vi "Advance Settings UI.vi"(0 "Advance Setting In":T1={"Prepare"={"Power Test Board.Voltage Level (V)"=0.0, "Power Test Board.Current Limit (A)"=0.0, "Fgen Voltage to Current Ratio"=1.0, "Fgen.Sample Rate (Sample/s)"=1.0}, "Stimulus And Measure"={"Fgen.Offset (V)"=0.0}} {"Stimulus And Measure"."Fgen.Offset (V)" min=1.0 format="%#_6p"; "Prepare"."Power Test Board.Current Limit (A)" min=1.0 format="%#_6p"; "Prepare"."Power Test Board.Voltage Level (V)" min=1.0 format="%#_6p"; "Prepare"."Fgen.Sample Rate (Sample/s)" min=1.0 format="%#_6p"; "Prepare"."Fgen Voltage to Current Ratio" min=1.0 format="%#_6p"}, 11 "error in (no error)":errorcluster) -> (4 "Advance Setting Out":T1={"Prepare"={"Power Test Board.Voltage Level (V)"=0.0, "Power Test Board.Current Limit (A)"=0.0, "Fgen Voltage to Current Ratio"=1.0, "Fgen.Sample Rate (Sample/s)"=1.0}, "Stimulus And Measure"={"Fgen.Offset (V)"=0.0}} {"Stimulus And Measure"."Fgen.Offset (V)" min=1.0 format="%#_6p"; "Prepare"."Power Test Board.Current Limit (A)" min=1.0 format="%#_6p"; "Prepare"."Power Test Board.Voltage Level (V)" min=1.0 format="%#_6p"; "Prepare"."Fgen.Sample Rate (Sample/s)" min=1.0 format="%#_6p"; "Prepare"."Fgen Voltage to Current Ratio" min=1.0 format="%#_6p"}, 15 "error out":errorcluster)   [LabVIEW 2020, in "LDO Load Transient_AWG.lvlib"]
uses:
  LDO Load Transient_AWG.lvlib
  Typedefs/Advance Settings.ctl
  Typedefs/Adv Settings Setup Instr.ctl
  Typedefs/Adv Settings Stimulus and Measure.ctl
  <vilib>/Utility/error.llb/DialogType.ctl
  <userlib>/_Soliton/Measurement Suite/Reusables/Queue Driver/Plugin Queue Driver.lvlib
  <userlib>/_Soliton/Measurement Suite/Reusables/Plugin Common/Plugin Common.lvlib
panel:
  in  "Current Limit (A)":dbl=0.1 min=1.0 format="%#_6p"
  in  "Voltage Level (V)":dbl=6.0 min=1.0 format="%#_6p"
  in  "Offset (V)":dbl min=1.0 format="%#_6p"
  in  "Sample Rate (Sample/s)":dbl=20000000.0 min=1.0 format="%#_6p"
  in  "Fgen Voltage to Current Ratio":dbl=1.0 min=1.0 format="%#_6p"
  in  "CLOSE":bool
  in  "Panel Close":bool
  out "Banner":picture caption="Advance Settings"
  # "Power Test Board"
  # "Fgen"
  # "Fgen"
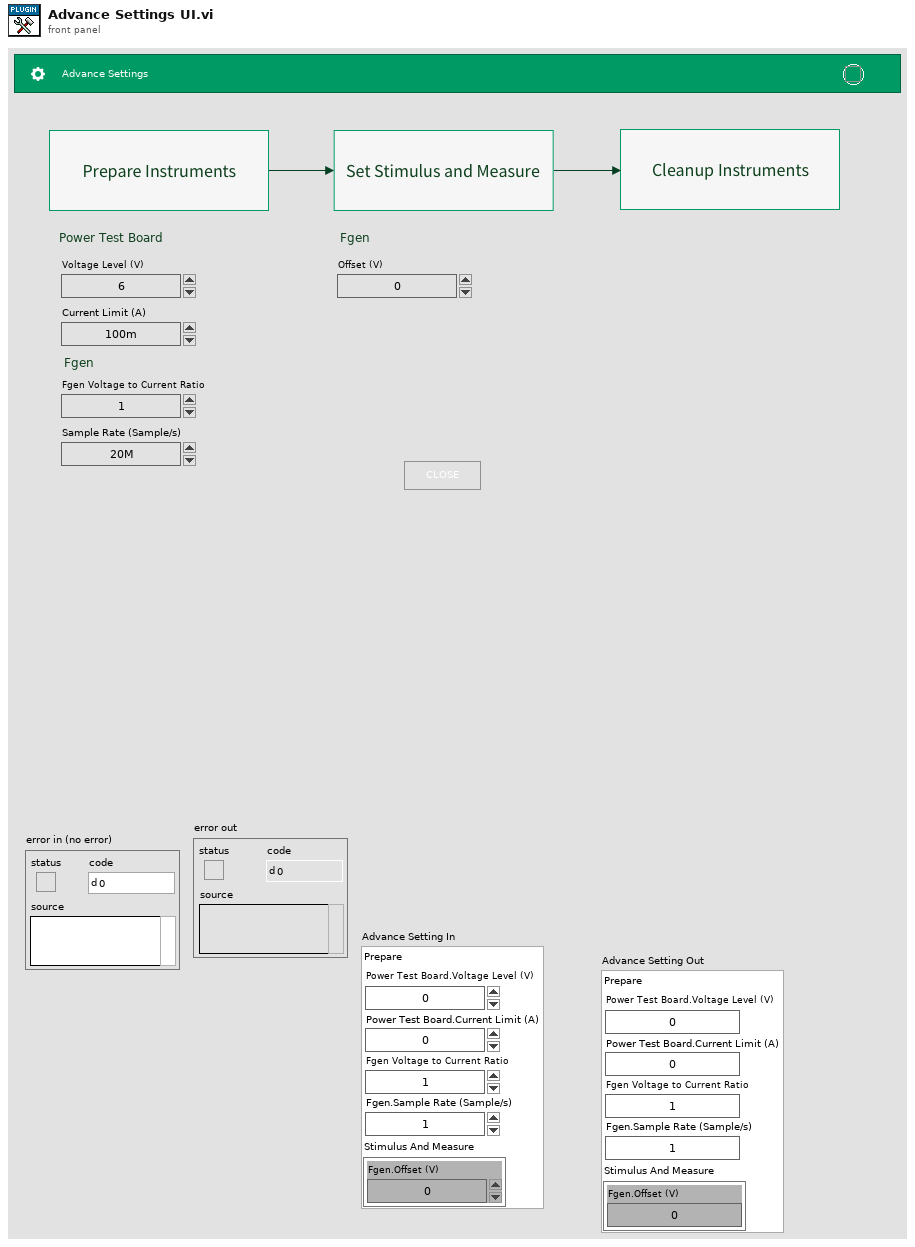
[diagram p1: front panel]
types:
  T1 = typedef "LDO Load Transient_AWG.lvlib/Advance Settings.ctl" = cluster{"Prepare":T2, "Stimulus And Measure":T3}
  T2 = typedef "LDO Load Transient_AWG.lvlib/Adv Settings Setup Instr.ctl" = cluster{"Power Test Board.Voltage Level (V)":dbl, "Power Test Board.Current Limit (A)":dbl, "Fgen Voltage to Current Ratio":dbl, "Fgen.Sample Rate (Sample/s)":dbl}
  T3 = typedef "LDO Load Transient_AWG.lvlib/Adv Settings Stimulus and Measure.ctl" = cluster{"Fgen.Offset (V)":dbl}
  T4 = typedef "DialogType.ctl" = u16
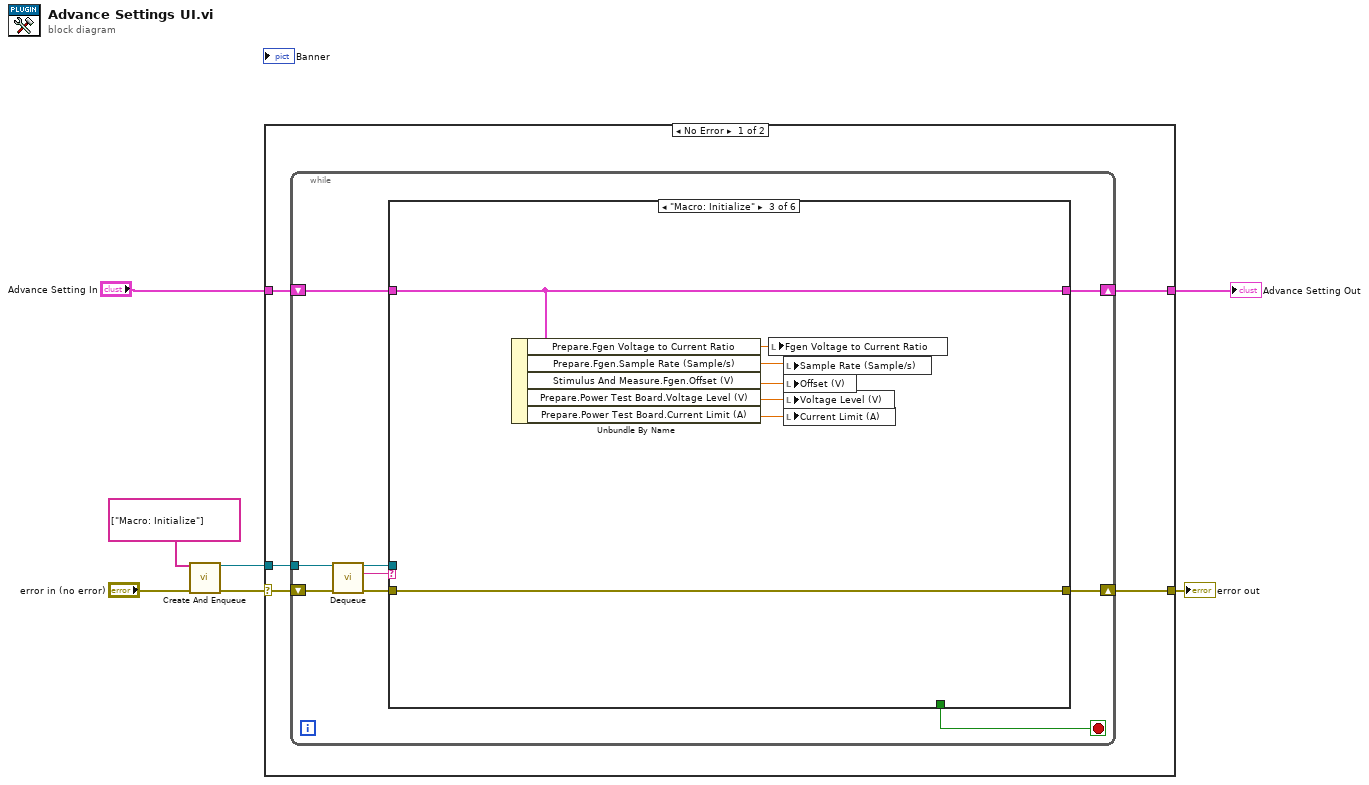
[diagram p0: block diagram]
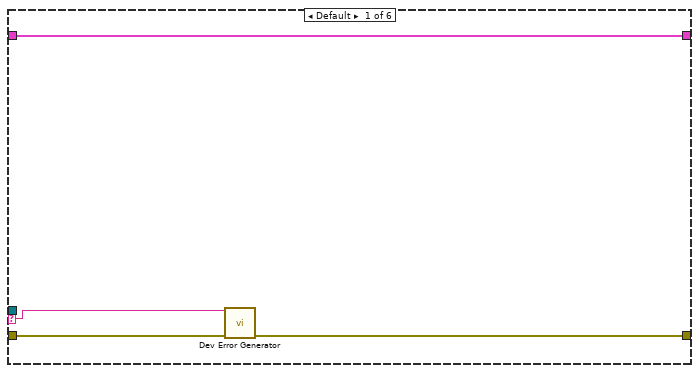
[diagram p2: hidden frame]
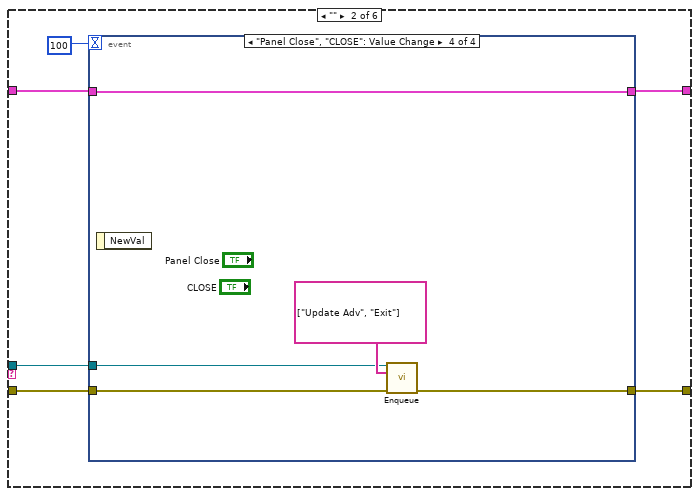
[diagram p3: hidden frame]
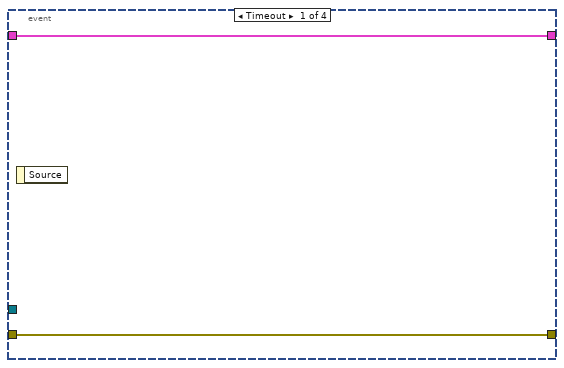
[diagram p4: hidden frame]
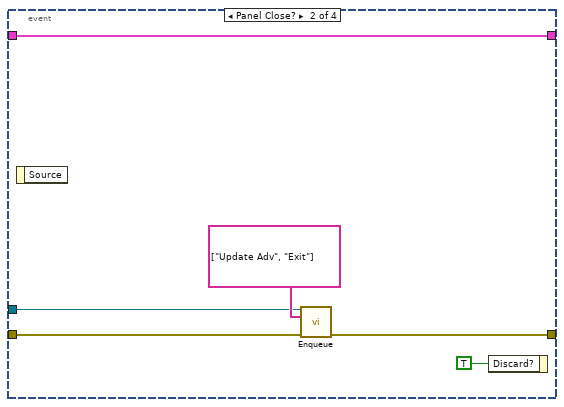
[diagram p5: hidden frame]
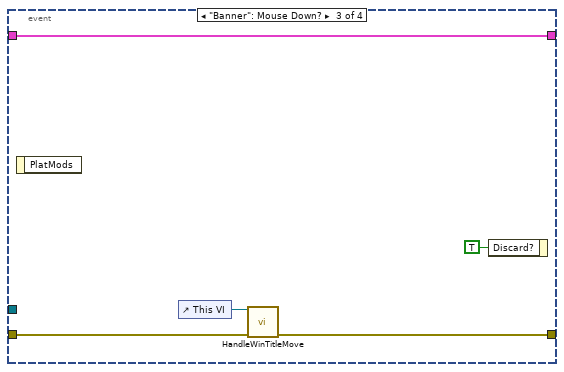
[diagram p6: hidden frame]
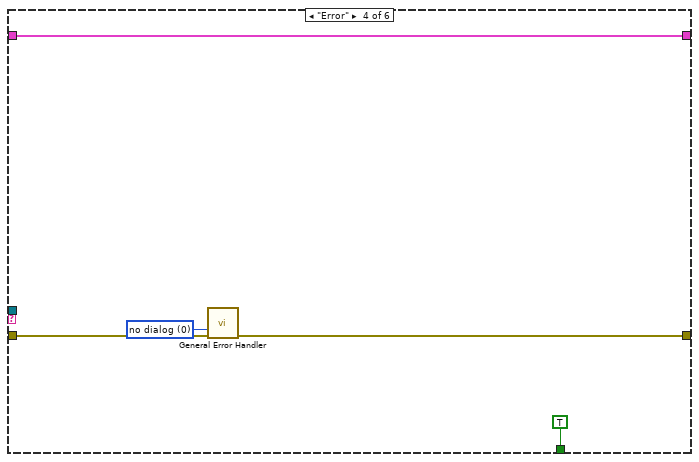
[diagram p7: hidden frame]
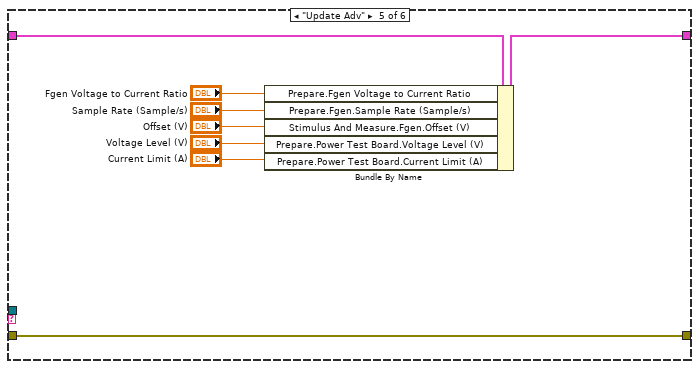
[diagram p8: hidden frame]
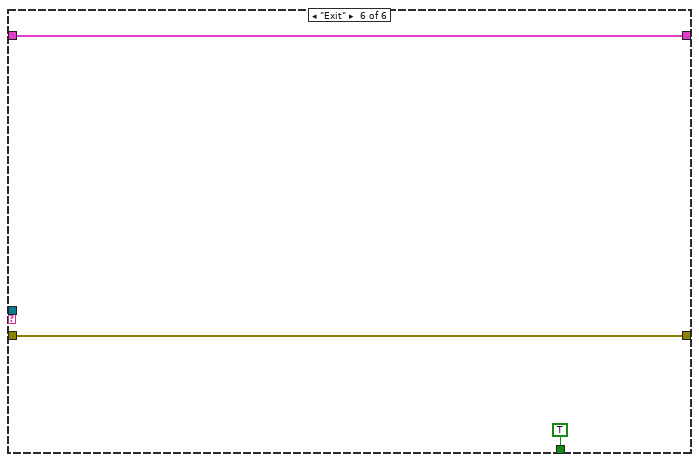
[diagram p9: hidden frame]
diagram:
  n1 = call <userlib>:"Create And Enqueue.vi"("Initial States"=string[] ["Macro: Initialize"], "error in (no error)"="error in (no error)") -> ("Queue out"=w4:refnum<queue>, "error out"=w5:errorcluster)  [unwired: 12 in]
  n2 = case shown="No Error" w5 {
    selector: w5 -> [w8 w74]
    tunnel: [w12 w74] -> w7
    tunnel: "Advance Setting In" -> [w11 w73]
    tunnel: [w10 w73] -> w1
    tunnel: w4 -> [w9 _]
    frame No Error {
      n3 = while {
        tunnel: w9 -> [w18]
        shift-right: [w19] -> w10
        shift-left: w11 -> [w20]
        shift-right: [w21] -> w12
        shift-left: w8 -> [w17]
        stop <- w14 stop-if-true
        n4 = call <userlib>:"Dequeue.vi"("Queue in"=w18, "error in (no error)"=w17) -> ("Queue out"=w13:refnum<queue>, "Dequeued State"=w15:string, "error out"=w16:errorcluster)  [unwired: 11 in]
        n5 = case shown="\"Macro: Initialize\"" w15 {
          selector: w15 -> [w22 _ _ _ _ _]
          tunnel: [w24 w31 w56 w59 w69 w72] -> w21
          tunnel: w20 -> [w25 w30 w55 w61 w67 w71]
          tunnel: [w25 w29 w55 w61 w68 w71] -> w19
          tunnel: w16 -> [w23 w28 w56 w58 w69 w72]
          tunnel: [_ _ _ TRUE _ TRUE ("Discard?")] -> w14
          tunnel: w13 -> [_ w26 _ _ _ _]
          frame Default {
            n6 = call <userlib>:"Dev Error Generator.vi"("State"=w22, "error in (no error)"=w23) -> ("error out"=w24:errorcluster)  [unwired: 13 in]
          }
          frame "" {
            n7 = event shown="[3] \"Panel Close\", \"CLOSE\": Value Change" {
              selector: _ -> [_ _ _ _]
              dyn-events: _ -> [_ _ _ _]
              timeout: 100 -> [_ _ _ _]
              tunnel: w28 -> [w33 w35 w41 w46]
              tunnel: [w33 w36 w42 w47] -> w31
              tunnel: w30 -> [w32 w39 w44 w49]
              tunnel: [w32 w39 w44 w49] -> w29
              tunnel: w26 -> [_ w34 _ w45]
              event Timeout {
                n8 = event-data() -> ()  [unwired: 1 in, 1 out]
              }
              event Panel Close? {
                n9 = event-data() -> ()  [unwired: 1 in, 1 out]
                n10 = call <userlib>:"Enqueue.vi"("Queue in"=w34, "States"=string[] ["Update Adv", "Exit"] ("Initial States"), "error in (no error)"=w35) -> ("error out"=w36:errorcluster)  [unwired: 11 in, 1 out]
                n11 = event-data("Discard?"=TRUE) -> ()  [unwired: 1 in, 1 out]
              }
              event "Banner": Mouse Down? {
                n12 = event-data() -> ()  [unwired: 1 in, 1 out]
                n13 = control-ref of="This VI"() -> (w40:refnum<vi>)
                n14 = call "HandleWinTitleMove.vi"("VI in"=w40, "error in (no error)"=w41) -> ("error out"=w42:errorcluster)  [unwired: 12 in, 1 out]
                n15 = event-data("Discard?"=TRUE) -> ()  [unwired: 1 in, 1 out]
              }
              event "Panel Close", "CLOSE": Value Change {
                n16 = event-data() -> ()  [unwired: 1 in, 1 out]
                n17 = call <userlib>:"Enqueue.vi"("Queue in"=w45, "States"=string[] ["Update Adv", "Exit"] ("Initial States"), "error in (no error)"=w46) -> ("error out"=w47:errorcluster)  [unwired: 11 in, 1 out]
              }
            }
          }
          frame "Macro: Initialize" {
            n18 = Unbundle By Name(w55) -> ("Prepare.Fgen Voltage to Current Ratio"=w54:dbl, "Prepare.Fgen.Sample Rate (Sample/s)"=w53:dbl, "Stimulus And Measure.Fgen.Offset (V)"=w52:dbl, "Prepare.Power Test Board.Voltage Level (V)"=w51:dbl, "Prepare.Power Test Board.Current Limit (A)"=w50:dbl)
            n19 = local write "Fgen Voltage to Current Ratio"(w54) -> ()
            n20 = local write "Sample Rate (Sample/s)"(w53) -> ()
            n21 = local write "Offset (V)"(w52) -> ()
            n22 = local write "Voltage Level (V)"(w51) -> ()
            n23 = local write "Current Limit (A)"(w50) -> ()
          }
          frame "Error" {
            w60 = T4 0 items=["no dialog", "OK message", "continue or stop message", "OK message + warnings", "continue/stop + warnings"] ("type of dialog (OK msg:1)")
            n24 = call <vilib>:"General Error Handler.vi"("type of dialog (OK msg:1)"=w60, "error in (no error)"=w58) -> ("error out"=w59:errorcluster)  [unwired: 9 in, 4 out]
          }
          frame "Update Adv" {
            n25 = Bundle By Name(cluster=w67, "Prepare.Fgen Voltage to Current Ratio"="Fgen Voltage to Current Ratio", "Prepare.Fgen.Sample Rate (Sample/s)"="Sample Rate (Sample/s)", "Stimulus And Measure.Fgen.Offset (V)"="Offset (V)", "Prepare.Power Test Board.Voltage Level (V)"="Voltage Level (V)", "Prepare.Power Test Board.Current Limit (A)"="Current Limit (A)") -> (w68:T1)
          }
          frame "Exit" {
          }
        }
      }
    }
    frame Error {
    }
  }
  "error out" <- w7
  "Advance Setting Out" <- w1
